vi "Demo - Shortcuts - Pt1_ SubVI.vi"(11 "NumIn":i32) -> (3 "NumOut":i32)   [LabVIEW 2020]
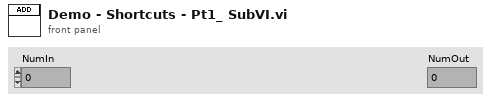
[diagram p1: front panel]
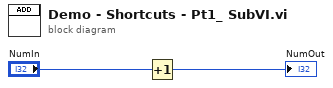
[diagram p0: block diagram]
diagram:
  n1 = Increment(x="NumIn") -> (x+1=→"NumOut":i32)
